vi "aft_xmpl_Delay Waveform.vi"(10 "delay (sec)":dbl, 11 "input":waveform(dbl)) -> (3 "output":waveform(dbl))   [LabVIEW 2019]
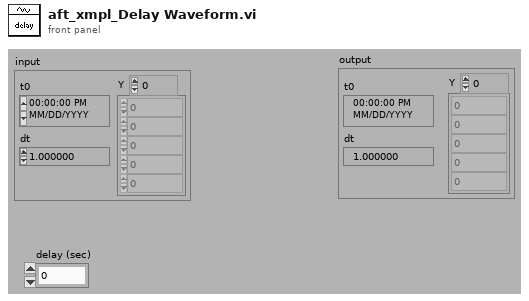
[diagram p1: front panel]
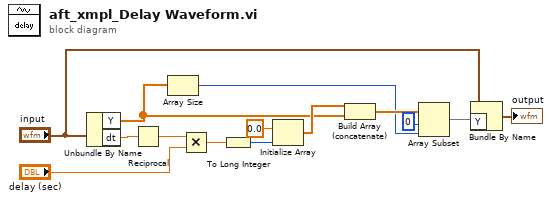
[diagram p0: block diagram]
diagram:
  n1 = Unbundle By Name("input") -> ("Y"=w1:dbl[], "dt"=w14:dbl)
  n2 = Reciprocal(x=w14) -> (1/x=w13:dbl)
  n3 = Array Size(array=w1) -> (size(s)=w7:i32)
  n4 = Multiply(x=w13, y="delay (sec)") -> (x*y=w11:dbl)
  n5 = To Long Integer(number=w11) -> (32bit integer=w10:i32)
  n6 = Initialize Array(0.0 ("element"), w10) -> (w2:dbl[])
  n7 = Build Array (concatenate)(w2, w1) -> (w8:dbl[])
  n8 = Array Subset(array=w8, index=0, length=w7) -> (w5:dbl[])
  n9 = Bundle By Name(cluster="input", "Y"=w5) -> (→"output":waveform(dbl))
